vi "Close.vi"(8 "error in (no error)":errorcluster, 11 "uService Template in":refnum<class "Kasli Server.lvclass">) -> (0 "error out":errorcluster, 3 "uService Template out":refnum<class "Kasli Server.lvclass">)   [LabVIEW 2020, in "CIRCUS_uServices.lvlib" / "Kasli Server.lvlib" / "Kasli Server.lvclass"]
uses:
  Kasli Server.lvclass
  Kasli Server.lvclass/Kasli Server.ctl
  TALOS/TALOS_PPL.lvlibp/Father of all uServices/Father of all uServices/Father of all uServices.lvclass
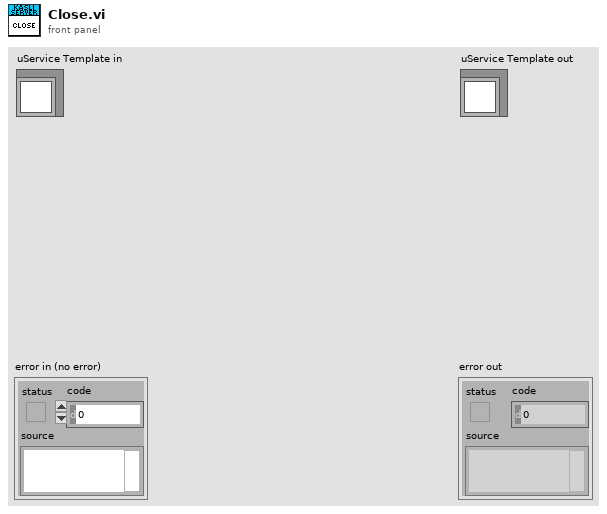
[diagram p1: front panel]
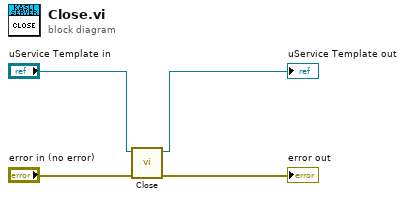
[diagram p0: block diagram]
diagram:
  n1 = call-parent "Close.vi"("error in (no error)"="error in (no error)", "uService Template in"="uService Template in") -> ("error out"=→"error out":errorcluster, "uService Template out"=→"uService Template out":refnum<class "Kasli Server.lvclass">)  [unwired: 8 in]
